vi "ParseAWGstring.vi"(2 "error constant":errorcluster, 3 "String":string) -> (0 "error out":errorcluster, 1 "Array":variant[](array[variant]))   [LabVIEW 2017]
panel:
  out "output cluster":T1
  in  "Channel cluster":T2(array[cluster])
  in  "Timing cluster":T3
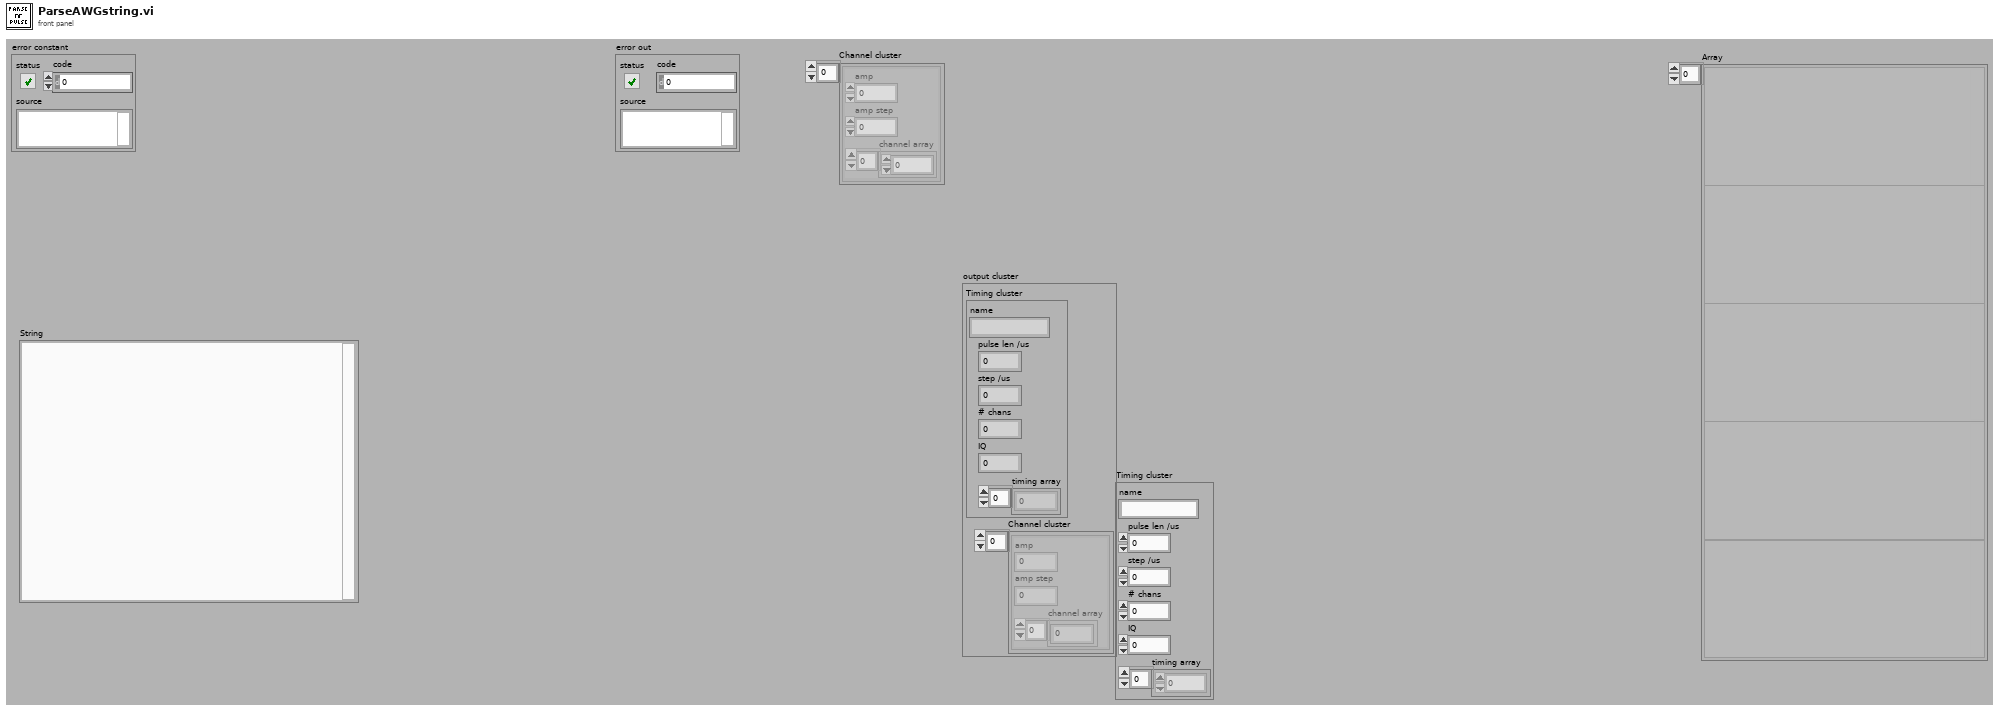
[diagram p1: front panel]
types:
  T1 = cluster{"Timing cluster":cluster{"name":string, "pulse len /us":dbl, "step /us":dbl, "# chans":i32, "IQ":i32, "timing array":dbl[]}, "Channel cluster":cluster{"amp":dbl, "amp step":dbl, "channel array":dbl[]}[]}
  T2 = cluster{"amp":dbl, "amp step":dbl, "channel array":dbl[]}[]
  T3 = cluster{"name":string, "pulse len /us":dbl, "step /us":dbl, "# chans":i32, "IQ":i32, "timing array":dbl[]}
  T4 = cluster{"Timing cluster 2":cluster{"name":string, "pulse len /us":dbl, "step /us":dbl, "# chans":i32, "IQ":i32, "timing array":dbl[]}, "Channel cluster 2":cluster{"amp":dbl, "amp step":dbl, "channel array":dbl[]}[]}
  T5 = cluster{"amp":dbl, "amp step":dbl, "array type (2D Dbl)":dbl[]}
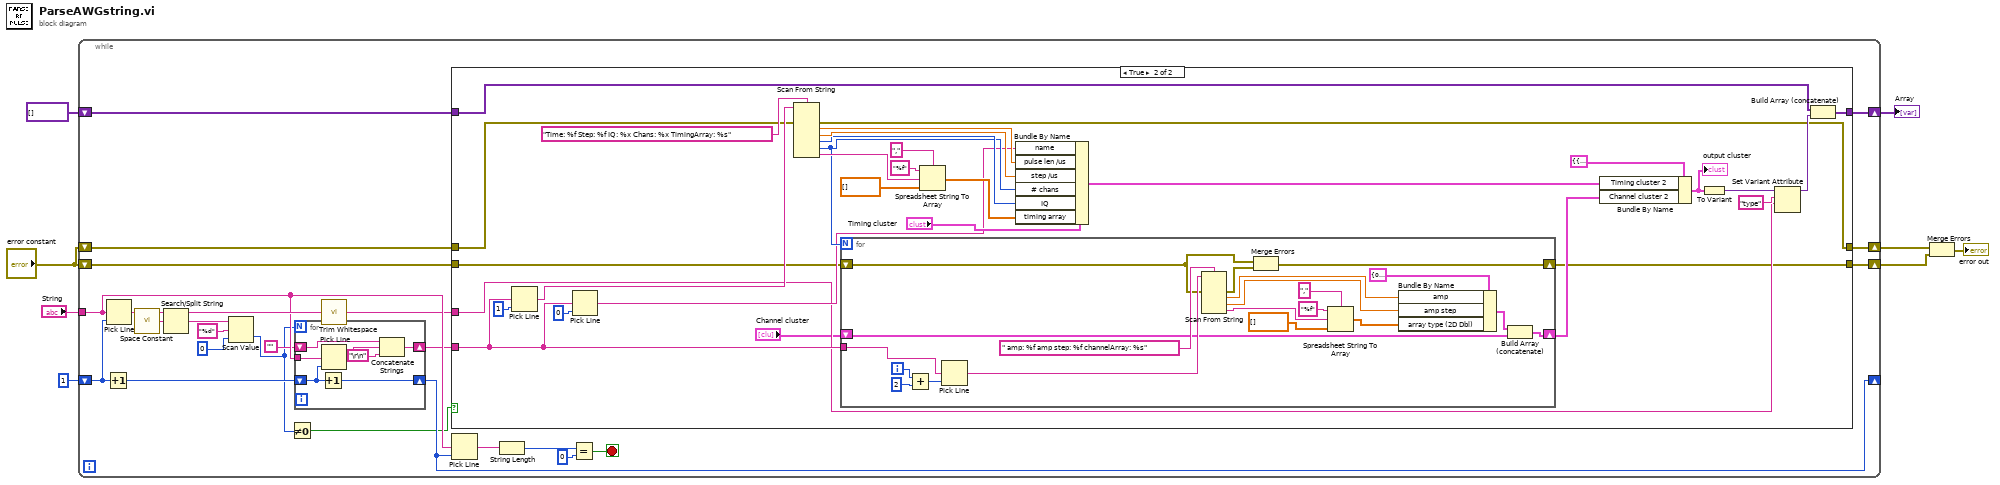
[diagram p0: block diagram]
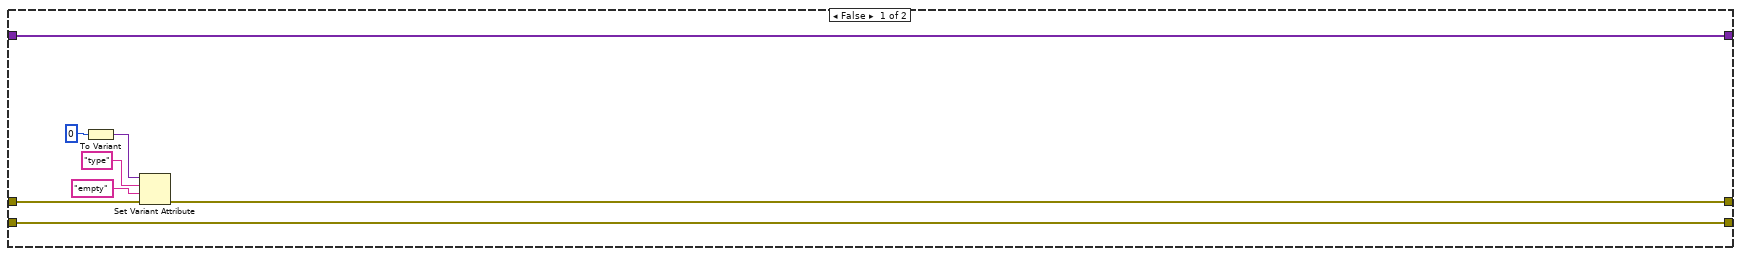
[diagram p2: hidden frame]
diagram:
  n1 = while {
    tunnel: "String" -> [w20]
    shift-right: [w21] -> _
    shift-left: 1 -> [w27]
    shift-right: [w14] -> w5
    shift-left: variant[] [] -> [w13]
    shift-right: [w11] -> w2
    shift-left: "error constant" -> [w12]
    shift-right: [w9] -> w3
    shift-left: "error constant" -> [w10]
    stop <- w22 stop-if-true
    n2 = Increment(x=w27) -> (x+1=w26:i32)
    n3 = Pick Line(multi-line string=w20, line index=w27) -> (output string=w33:string)  [unwired: 1 in]
    n4 = call <vilib>:"Space Constant.vi"() -> ("String"=w32:string)
    n5 = Search/Split String(string=w33, search string/char (-)=w32) -> (substring before match=w31:string, match + rest of string=w30:string)  [unwired: 1 in, 1 out]
    n6 = Scan Value(string=w30, format string="%d", default (0 dbl)=0) -> (value=w15:i32)  [unwired: 1 out]
    n7 = Not Equal To 0?(x=w15) -> (x != 0?=w16:bool)
    n8 = for {
      N: w15 -> [_]
      tunnel: w20 -> [w97]
      shift-right: [w99] -> w21
      shift-left: w26 -> [w98]
      shift-right: [w93] -> w19
      shift-left: "" -> [w96]
      n9 = Increment(x=w98) -> (x+1=w99:i32)
      n10 = Pick Line(multi-line string=w97, line index=w98) -> (output string=w95:string)  [unwired: 1 in]
      n11 = Concatenate Strings(w96, w95, "\r\n") -> (w93:string)
    }
    n12 = call <vilib>:"Trim Whitespace.vi"("string"=w31) -> ("trimmed string"=w17:string)  [unwired: 1 in]
    n13 = case shown="True" w16 {
      tunnel: w19 -> [_ w72]
      tunnel: w17 -> [_ w50]
      tunnel: [w37 w48] -> w14
      tunnel: w13 -> [w37 w47]
      tunnel: w12 -> [w34 w45]
      tunnel: [w34 w44] -> w11
      tunnel: w10 -> [w36 w43]
      tunnel: [w35 w42] -> w9
      frame False {
        n14 = To Variant(anything=0) -> (Variant=w40:variant)
        n15 = Set Variant Attribute(Variant=w40, name="type", value="empty" ("name"), error in=w36) -> (error out=w35:errorcluster)  [unwired: 2 out]
      }
      frame True {
        n16 = Pick Line(multi-line string=w72, line index=1) -> (output string=w71:string)  [unwired: 1 in]
        n17 = Pick Line(multi-line string=w72, line index=0) -> (output string=w57:string)  [unwired: 1 in]
        n18 = Scan From String(format string="Time: %f Step: %f IQ: %x Chans: %x TimingArray: %s", input string=w71, error in=w43) -> (error out=w42:errorcluster, output 1=w69:dbl, output 2=w70:dbl, output 3=w60:u32, output 4=w59:u32, output 5=w62:string)  [unwired: 6 in, 2 out]
        n19 = for {
          N: w59 -> [_]
          shift-right: [w80] -> w54
          shift-left: "Channel cluster" -> [w81]
          tunnel: w72 -> [w91]
          shift-right: [w73] -> w44
          shift-left: w45 -> [w74]
          i -> [w90]
          n20 = Add(x=w90, y=2) -> (x+y=w89:i32)
          n21 = Pick Line(multi-line string=w91, line index=w89) -> (output string=w87:string)  [unwired: 1 in]
          n22 = Scan From String(format string=" amp: %f amp step: %f channelArray: %s", input string=w87, error in=w74) -> (error out=w75:errorcluster, output 1=w76:dbl, output 2=w77:dbl, output 3=w83:string)  [unwired: 4 in, 2 out]
          n23 = Merge Errors(w74, w75) -> (w73:errorcluster)
          n24 = Spreadsheet String To Array(delimiter (Tab)=",", format string="%f", spreadsheet string=w83, array type (2D Dbl)=dbl[] []) -> (array=w78:dbl[])
          n25 = Bundle By Name(cluster=T5 {"amp"=0.0, "amp step"=0.0, "array type (2D Dbl)"=[]} ("freq cluster"), "amp"=w76, "amp step"=w77, "array type (2D Dbl)"=w78) -> (w79:T5)
          n26 = Build Array (concatenate)(w79, w81) -> (w80:T2)
        }
        n27 = Spreadsheet String To Array(delimiter (Tab)=",", format string="%f", spreadsheet string=w62, array type (2D Dbl)=dbl[] []) -> (array=w58:dbl[])
        n28 = Bundle By Name(cluster="Timing cluster", "name"=w57, "pulse len /us"=w69, "step /us"=w70, "# chans"=w59, "IQ"=w60, "timing array"=w58) -> (w55:T3)
        n29 = Bundle By Name(cluster=T4 {"Timing cluster 2"={"name"="", "pulse len /us"=0.0, "step /us"=0.0, "# chans"=0, "IQ"=0, "timing array"=[]}, "Channel cluster 2"=[]} ("RF pulse cluster"), "Timing cluster 2"=w55, "Channel cluster 2"=w54) -> (w53:T4)
        "output cluster" <- w53
        n30 = To Variant(anything=w53) -> (Variant=w52:variant)
        n31 = Set Variant Attribute(Variant=w52, name="type", value=w50) -> (Variant out=w46:variant)  [unwired: 1 in, 2 out]
        n32 = Build Array (concatenate)(w47, w46) -> (w48:variant[])
      }
    }
    n33 = Pick Line(multi-line string=w20, line index=w21) -> (output string=w25:string)  [unwired: 1 in]
    n34 = String Length(string=w25) -> (length=w24:i32)
    n35 = Equal?(x=w24, y=0) -> (x = y?=w22:bool)
  }
  "Array" <- w5
  n36 = Merge Errors(w3, w2) -> (→"error out":errorcluster)
